vi "series_top_coord.vi"(8 "error in (no error)":errorcluster, 10 "ROI Descriptor":T1 {"Contours"."Type" items=["No Selection", "Point", "Line", "Rectangle", "Oval", "Polygon", "Freehand Region", "Annulus", "Unused2", "Unused3", "Broken Line", "Freehand Line", "Rotated Rectangle"]}, 11 "New Image":T3(plugin-control)) -> (0 "error out":errorcluster, 3 "Co Ordinate System":T2)   [LabVIEW 2019, in "Algorithm.lvclass"]
uses:
  FrameworkOverrides/Algorithm.lvclass
  <vilib>/vision/NI_Vision_Development_Module.lvlib
panel:
  out "Array 2":bool[](array[boolean])
  out "Area":dbl[](array[numeric])
  out "Image 2":T3(plugin-control)
  out "X Coord":dbl[](array[numeric])
  out "Number of Particles":i32
  out "Y Coord":dbl[](array[numeric])
  out "x-y":u64
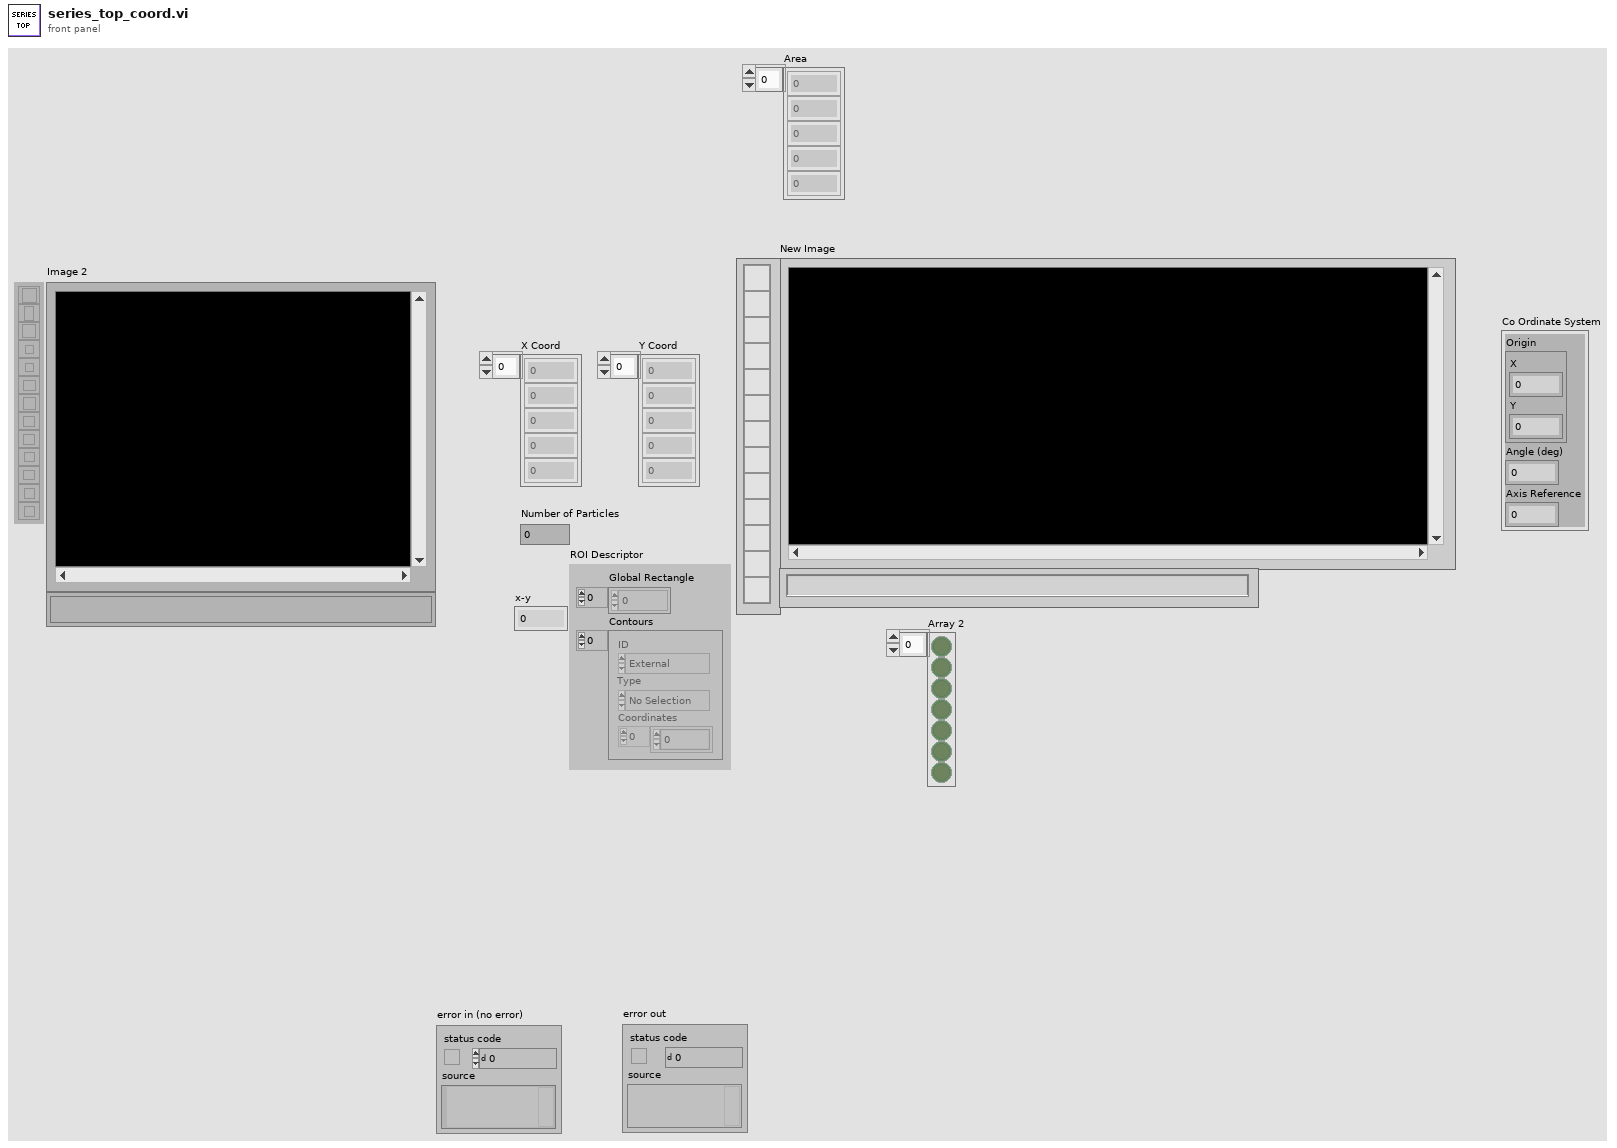
[diagram p1: front panel]
types:
  T1 = typedef "ROI Descriptor" = cluster{"Global Rectangle":i32[], "Contours":cluster{"ID":enum32{"External", "Internal"}, "Type":u32, "Coordinates":i32[]}[]}
  T2 = cluster{"Origin":cluster{"X":sgl, "Y":sgl}, "Angle (deg)":sgl, "Axis Reference":u32}
  T3 = typedef "IMAQ Image.ctl" = refnum<image>
  T4 = typedef "Particle Parameters" = i32
  T5 = cluster{"Measurement Parameter":T4, "Range Lower Value":dbl, "Range Upper Value":dbl, "Range":bool, "Measurement Type":bool}[]
  T6 = typedef "Image Type" = u32
  T7 = typedef "IMAQ Rectangle" = cluster{"Left":i32, "Top":i32, "Right":i32, "Bottom":i32, "Rotation":dbl}
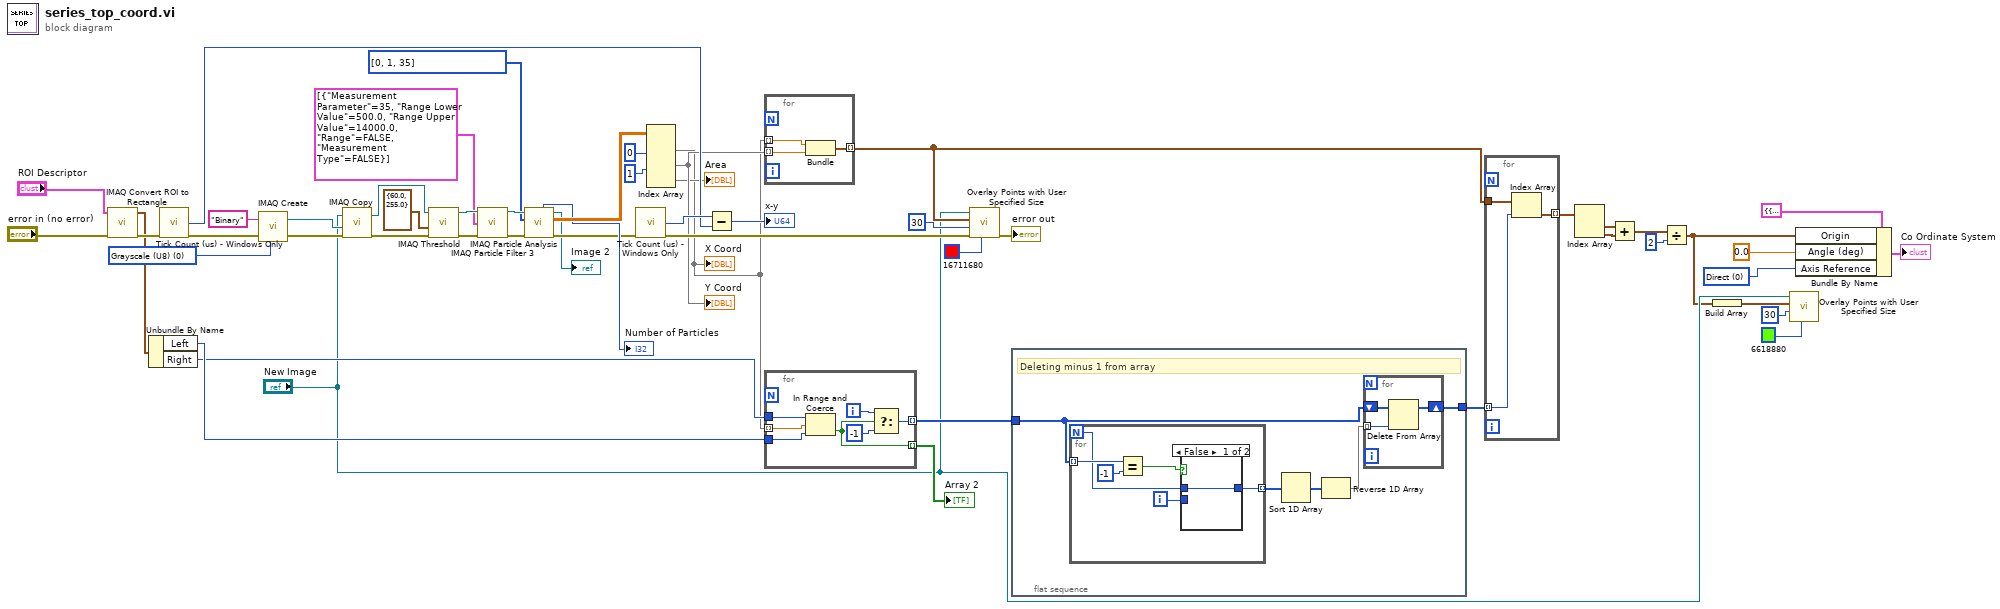
[diagram p0: block diagram]
diagram:
  w7 = u32 0 items=["Direct", "Indirect"] ("Axis Reference")
  w46 = T4[] [0, 1, 35] items=["Center of Mass X", "Center of Mass Y", "First Pixel X", "First Pixel Y", "Bounding Rect Left", "Bounding Rect Top", "Bounding Rect Right", "Bounding Rect Bottom", "Max Feret Diameter Start X", "Max Feret Diameter Start Y", "Max Feret Diameter End X", "Max Feret Diameter End Y", "Max Horiz. Segment Length Left", "Max Horiz. Segment Length Right", "Max Horiz. Segment Length Row", "-", "Bounding Rect Width", "Bounding Rect Height", "Bounding Rect Diagonal", "Perimeter", "Convex Hull Perimeter", "Holes' Perimeter", "Max Feret Diameter", "Equivalent Ellipse Major Axis", "Equivalent Ellipse Minor Axis", "Equivalent Ellipse Minor Axis (Feret)", "Equivalent Rect Long Side", "Equivalent Rect Short Side", "Equivalent Rect Diagonal", "Equivalent Rect Short Side (Feret)", "Average Horiz. Segment Length", "Average Vert. Segment Length", "Hydraulic Radius", "Waddel Disk Diameter", "-", "Area", "Holes' Area", "Particle & Holes' Area", "Convex Hull Area", "Image Area", "-", "Number of Holes", "Number of Horiz. Segments", "Number of Vert. Segments", "-", "Orientation", "Max Feret Diameter Orientation", "-", "% Area/Image Area", "% Area/(Particle & Holes' Area)", "Ratio of Equivalent Ellipse Axes", "Ratio of Equivalent Rect Sides", "-", "Elongation Factor", "Compactness Factor", "Heywood Circularity Factor", "Type Factor", "-", "Sum X", "Sum Y", "Sum XX", "Sum XY", "Sum YY", "Sum XXX", "Sum XXY", "Sum XYY", "Sum YYY", "-", "Moment of Inertia XX", "Moment of Inertia XY", "Moment of Inertia YY", "Moment of Inertia XXX", "Moment of Inertia XXY", "Moment of Inertia XYY", "Moment of Inertia YYY", "Norm. Moment of Inertia XX", "Norm. Moment of Inertia XY", "Norm. Moment of Inertia YY", "Norm. Moment of Inertia XXX", "Norm. Moment of Inertia XXY", "Norm. Moment of Inertia XYY", "Norm. Moment of Inertia YYY", "Hu Moment 1", "Hu Moment 2", "Hu Moment 3", "Hu Moment 4", "Hu Moment 5", "Hu Moment 6", "Hu Moment 7"] ("Pixel Measurements")
  w52 = T6 0 items=["Grayscale (U8)", "Grayscale (I16)", "Grayscale (SGL)", "Complex (CSG)", "RGB (U32)", "HSL (U32)", "RGB (U64)", "Grayscale (U16)"] ("Image Type")
  n1 = call "IMAQ Convert ROI to Rectangle"("error in (no error)"="error in (no error)", "ROI Descriptor"="ROI Descriptor") -> ("error out"=w26:errorcluster, "Rectangle"=w25:T7)  [unwired: 7 in]
  n2 = Unbundle By Name(w25) -> ("Left"=w24:i32, "Right"=w23:i32)
  n3 = call "Tick Count (us) - Windows Only.vi"("error in (no error)"=w26) -> ("micorsecond timer value"=w35:u64, "error out"=w30:errorcluster)  [unwired: 13 in]
  n4 = call "IMAQ Create"("Image Name"="Binary", "Image Type"=w52, "error in (no error)"=w30) -> ("New Image"=w51:T3, "error out"=w37:errorcluster)  [unwired: 2 in]
  n5 = call "IMAQ Copy"("error in (no error)"=w37, "Image Dst"=w51, "Image Src"="New Image") -> ("error out"=w38:errorcluster, "Image Dst Out"=w45:T3)  [unwired: 3 in]
  n6 = call "IMAQ Threshold"("error in (no error)"=w38, "Range"=cluster{"Lower value":sgl, "Upper value":sgl} {"Lower value"=60.0, "Upper value"=255.0}, "Image Src"=w45) -> ("error out"=w50:errorcluster, "Image Dst Out"=w49:T3)  [unwired: 7 in]
  n7 = call "IMAQ Particle Filter 3"("Image Src"=w49, "Selection Values"=T5 [{"Measurement Parameter"=35, "Range Lower Value"=500.0, "Range Upper Value"=14000.0, "Range"=FALSE, "Measurement Type"=FALSE}], "error in (no error)"=w50) -> ("Image Dst Out"=w48:T3, "error out"=w47:errorcluster)  [unwired: 10 in, 1 out]
  n8 = call "IMAQ Particle Analysis"("error in (no error)"=w47, "Pixel Measurements"=w46, "Image"=w48) -> ("error out"=w31:errorcluster, "Particle Measurements (Pixels)"=w43:dbl[][], "Image Out (duplicate)"=→"Image 2":T3, "Number of Particles"=→"Number of Particles":i32)  [unwired: 3 in, 2 out]
  n9 = call "Tick Count (us) - Windows Only.vi"("error in (no error)"=w31) -> ("micorsecond timer value"=w36:u64, "error out"=w34:errorcluster)  [unwired: 13 in]
  n10 = Index Array(array=w43, index (col) #1=0 ("disabled index (col)"), index (col) #2=1 ("index (col)")) -> (element #1=w22:dbl[], element #2=w29:dbl[], element #3=→"Area":dbl[])  [unwired: 4 in]
  "X Coord" <- w22
  "Y Coord" <- w29
  n11 = Subtract(x=w36, y=w35) -> (x-y=→"x-y":u64)
  n12 = for {
    tunnel: w22 -> [w57] mode=indexing
    tunnel: w29 -> [w56] mode=indexing
    tunnel: [w55] -> w20 mode=indexing
    n13 = Bundle("Numeric"=w57, "Numeric"=w56) -> (w55:cluster{"Numeric":dbl, "Numeric":dbl})  [unwired: 1 in]
  }
  n14 = for {
    tunnel: w24 -> [w58]
    tunnel: w23 -> [w59]
    tunnel: w22 -> [w64] mode=indexing
    tunnel: [w63] -> w19 mode=indexing
    tunnel: [w60] -> w21 mode=indexing
    i -> [w62]
    n15 = In Range and Coerce(upper limit=w59, x=w64, lower limit=w58) -> (In Range?=w60:bool)  [unwired: 1 out]
    n16 = Select(t=w62, s=w60, f=-1) -> (s? t:f=w63:i32)
  }
  "Array 2" <- w21
  n17 = call "Overlay Points with User Specified Size.vi"("Color"=u32 16711680, "error in"=w34, "Point Diameter (5)"=u32 30, "Points"=w20, "Image In"="New Image") -> ("error out"=→"error out":errorcluster)  [unwired: 5 in, 1 out]
  n18 = flat-sequence {
    tunnel: w19 -> [w66]
    tunnel: [w65] -> w18
    frame #0 {
      # "Deleting minus 1 from array"
      n19 = for {
        N -> [w74]
        tunnel: w66 -> [w78] mode=indexing
        tunnel: [w75] -> w67 mode=indexing
        i -> [w76]
        n20 = Equal?(x=w78, y=-1) -> (x = y?=w77:bool)
        n21 = case shown="False" w77 {
          tunnel: w76 -> [_ w80]
          tunnel: [w79 w80] -> w75
          tunnel: w74 -> [w79 _]
          frame False {
          }
          frame True {
          }
        }
      }
      n22 = Sort 1D Array(array=w67) -> (sorted array=w69:i32[])
      n23 = Reverse 1D Array(array=w69) -> (reversed array=w68:i32[])
      n24 = for {
        tunnel: w68 -> [w71] mode=indexing
        shift-right: [w70] -> w65
        shift-left: w66 -> [w72]
        n25 = Delete From Array(array=w72, index=w71) -> (array with subset deleted=w70:i32[])  [unwired: 1 in, 1 out]
      }
    }
  }
  n26 = for {
    tunnel: w18 -> [w82] mode=indexing
    tunnel: w20 -> [w83]
    tunnel: [w81] -> w17 mode=indexing
    n27 = Index Array(array=w83, index=w82) -> (element=w81:cluster{"Numeric":dbl, "Numeric":dbl})
  }
  n28 = Index Array(array=w17) -> (element #1=w16:cluster{"Numeric":dbl, "Numeric":dbl}, element #2=w15:cluster{"Numeric":dbl, "Numeric":dbl})  [unwired: 2 in]
  n29 = Add(x=w16, y=w15) -> (x+y=w14:cluster{"Numeric":dbl, "Numeric":dbl})
  n30 = Divide(x=w14, y=2) -> (x/y=w5:cluster{"Numeric":dbl, "Numeric":dbl})
  n31 = Build Array(w5) -> (w10:cluster{"Numeric":dbl, "Numeric":dbl}[])
  n32 = call "Overlay Points with User Specified Size.vi"("Color"=u32 6618880, "Point Diameter (5)"=u32 30, "Points"=w10, "Image In"="New Image") -> ()  [unwired: 6 in, 2 out]
  n33 = Bundle By Name(cluster=T2 {"Origin"={"X"=0.0, "Y"=0.0}, "Angle (deg)"=0.0, "Axis Reference"=0} ("Coordinate System"), "Origin"=w5, "Angle (deg)"=sgl 0.0, "Axis Reference"=w7) -> (→"Co Ordinate System":T2)
